vi "Delay.vi"(2 "Delay, ms":u32, 5 "error in":errorcluster={"status"=FALSE, "code"=1073676294, "source"="VISA Read in CONEC-CC.lvclass:WriteReadSerialPort.vi->CONEC-CC.lvclass:Get Motion Time.vi->Stage Control 01.vi"}) -> (19 "error out":errorcluster={"status"=FALSE, "code"=1073676294, "source"="VISA Read in CONEC-CC.lvclass:WriteReadSerialPort.vi->CONEC-CC.lvclass:Get Motion Time.vi->Stage Control 01.vi"})   [LabVIEW 2018]
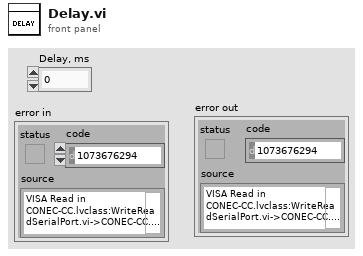
[diagram p1: front panel]
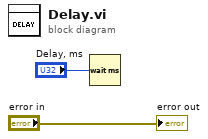
[diagram p0: block diagram]
diagram:
  n1 = Wait (ms)(milliseconds to wait="Delay, ms") -> ()  [unwired: 1 out]
  "error out" <- "error in"
